vi "Parse OSZICAR (Energies).vi"(8 "error in (no error)":errorcluster, 9 "Reference Energy/atom (pure Crystal) (eV)":dbl=-2.489625, 10 "# of Atoms":i32, 11 "OSZICAR File":path) -> (0 "Summary Values":string[](array[string])=["# Atoms", "Cell Volume (A^3)", "|C|"], 1 "Summary Headers":string[](array[string])=["# Atoms", "Cell Volume (A^3)", "|A| (Å)", "|B| (Å)", "|C| (Å)", "alpha (deg)", "beta (deg)", "gamma (deg)"], 2 "OSZICAR Raw":T1, 3 "Extracted Parameters":T3)   [LabVIEW 2010]
panel:
  out "OSZICAR data":T2(array[cluster]) {"Total Free Energy (eV)" format="%#_10g"}
  out "error out":errorcluster
  out "Bulk Formation Energies Array (eV)":dbl[](array[numeric])
  out "Ionic Relaxation Energies Array (eV)":dbl[](array[numeric])
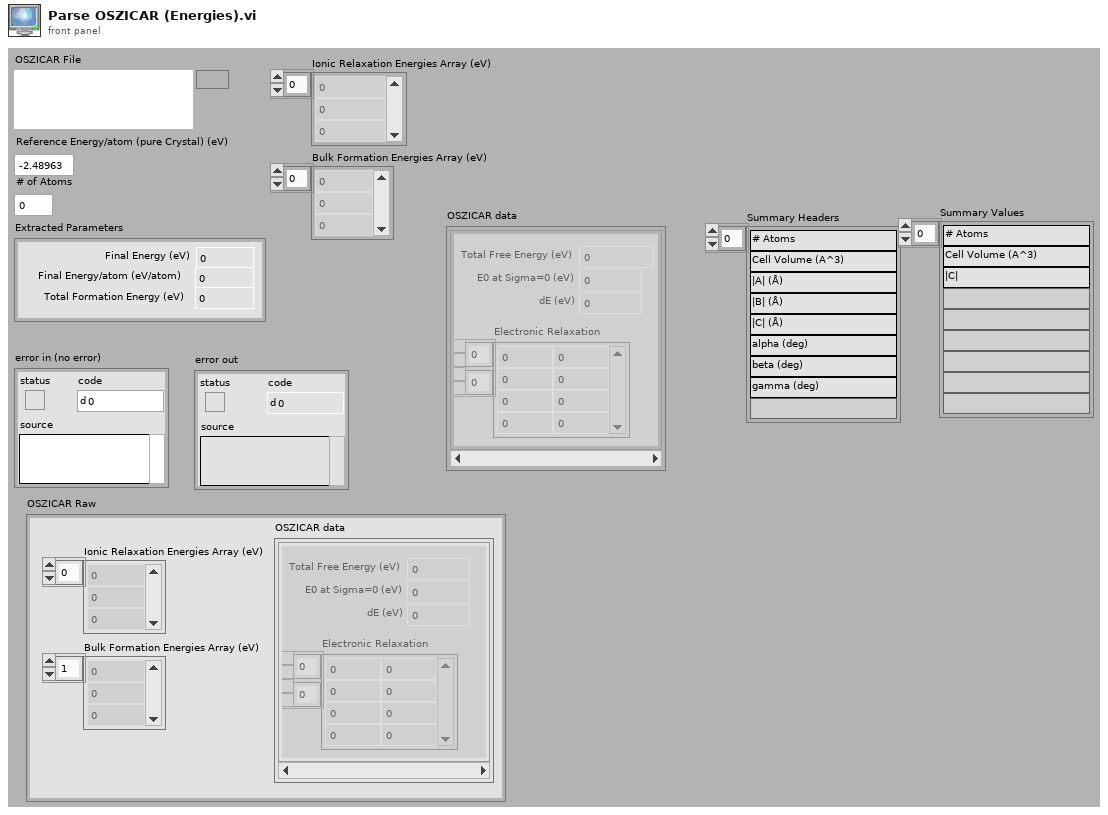
[diagram p1: front panel]
types:
  T1 = cluster{"OSZICAR data":cluster{"Total Free Energy (eV)":dbl, "E0 at Sigma=0 (eV)":dbl, "dE (eV)":dbl, "Electronic Relaxation":dbl[][]}[], "Ionic Relaxation Energies Array (eV)":dbl[], "Bulk Formation Energies Array (eV)":dbl[]}
  T2 = cluster{"Total Free Energy (eV)":dbl, "E0 at Sigma=0 (eV)":dbl, "dE (eV)":dbl, "Electronic Relaxation":dbl[][]}[]
  T3 = cluster{"Final Energy (eV)":dbl, "Final Energy/atom (eV/atom)":dbl, "Total Formation Energy (eV)":dbl}
  T4 = cluster{"Total Free Energy (eV)":dbl, "E0 at Sigma=0 (eV)":dbl, "dE (eV)":dbl, "Electronic Relaxation":dbl[][]}
  T5 = cluster{"OSZICAR data 2":cluster{"Total Free Energy (eV)":dbl, "E0 at Sigma=0 (eV)":dbl, "dE (eV)":dbl, "Electronic Relaxation":dbl[][]}[], dbl[], dbl[]}
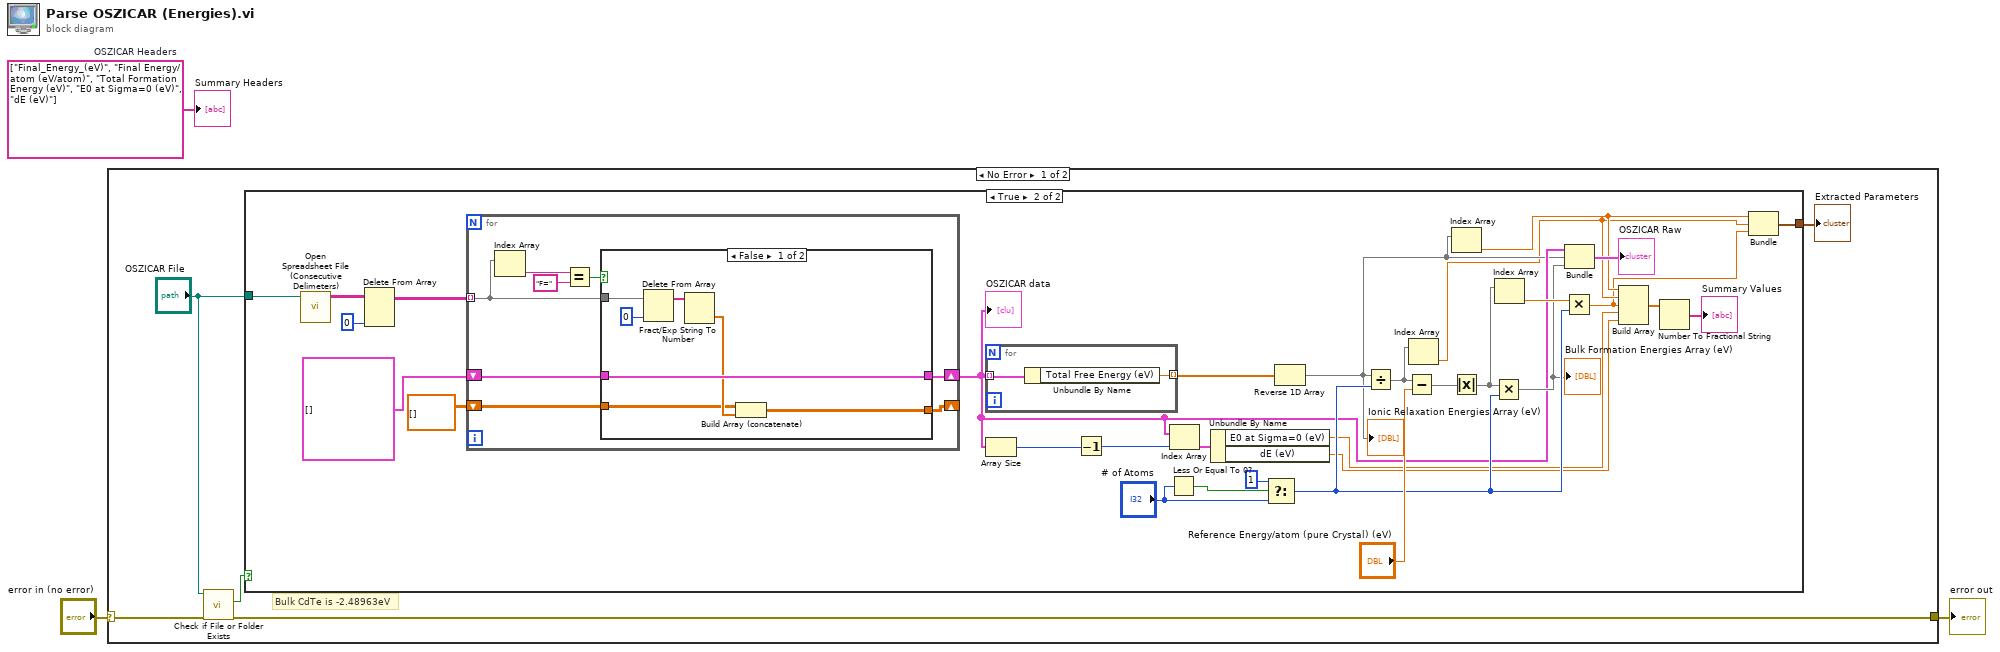
[diagram p0: block diagram]
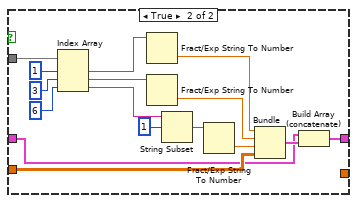
[diagram p3: hidden frame]
diagram:
  w1 = string[] ["Final_Energy_(eV)", "Final Energy/atom (eV/atom)", "Total Formation Energy (eV)", "E0 at Sigma=0 (eV)", "dE (eV)"]  # OSZICAR Headers
  n1 = case shown="No Error" "error in (no error)" {
    selector: "error in (no error)" -> [w5 w73]
    tunnel: [w4 w73] -> w2
    frame No Error {
      # "Bulk CdTe is -2.48963eV"
      n2 = call <vilib>:"Check if File or Folder Exists.vi"("error in (no error)"=w5, "path"="OSZICAR File") -> ("error out"=w4:errorcluster, "file or folder exists?"=w7:bool)  [unwired: 7 in, 1 out]
      n3 = case shown="True" w7 {
        tunnel: "OSZICAR File" -> [_ w29]
        tunnel: [_ w30] -> w6
        frame False {
        }
        frame True {
          n4 = call "Open Spreadsheet File (Consecutive Delimeters).vi"("File"=w29) -> ("Array"=w28:string[][])  [unwired: 9 in, 1 out]
          n5 = Delete From Array(array=w28, index (col)=0 ("disabled index (col)")) -> (array with subset deleted=w26:string[][])  [unwired: 2 in, 1 out]
          n6 = for {
            tunnel: w26 -> [w46] mode=indexing
            shift-right: [w45] -> _
            shift-left: dbl[][] [] -> [w44]
            shift-right: [w43] -> w20
            shift-left: T2 [] ("OSZICAR data 2") -> [w42]
            n7 = Index Array(array=w46) -> (element=w49:string)  [unwired: 1 in]
            n8 = Equal?(x=w49, y="F=") -> (x = y?=w47:bool)
            n9 = case shown="False" w47 {
              tunnel: w46 -> [w55 w64]
              tunnel: [w51 _] -> w45
              tunnel: w44 -> [w50 w69]
              tunnel: [w56 w67] -> w43
              tunnel: w42 -> [w56 w66]
              frame False {
                n10 = Delete From Array(array=w55, index=0) -> (array with subset deleted=w53:string[])  [unwired: 1 in, 1 out]
                n11 = Fract/Exp String To Number(string=w53) -> (number=w52:dbl[])  [unwired: 3 in, 1 out]
                n12 = Build Array (concatenate)(w50, w52) -> (w51:dbl[][])
              }
              frame True {
                n13 = Index Array(array=w64, index #1=1 ("index"), index #2=3 ("index"), index #3=6 ("index")) -> (element #1=w63:string, element #2=w61:string, element #3=w59:string)
                n14 = Fract/Exp String To Number(string=w63) -> (number=w62:dbl)  [unwired: 3 in, 1 out]
                n15 = Fract/Exp String To Number(string=w61) -> (number=w60:dbl)  [unwired: 3 in, 1 out]
                n16 = String Subset(string=w59, offset (0)=1) -> (substring=w58:string)  [unwired: 1 in]
                n17 = Fract/Exp String To Number(string=w58) -> (number=w57:dbl)  [unwired: 3 in, 1 out]
                n18 = Bundle(w62, w60, w57, w69) -> (w68:cluster{dbl, dbl, dbl, dbl[][]})  [unwired: 1 in]
                n19 = Build Array (concatenate)(w66, w68) -> (w67:T2)
              }
            }
          }
          "OSZICAR data" <- w20
          n20 = for {
            tunnel: w20 -> [w41] mode=indexing
            tunnel: [w40] -> w23 mode=indexing
            n21 = Unbundle By Name(w41) -> ("Total Free Energy (eV)"=w40:dbl)
          }
          n22 = Array Size(array=w20) -> (size(s)=w19:i32)
          n23 = Decrement(x=w19) -> (x-1=w18:i32)
          n24 = Less Or Equal To 0?(x="# of Atoms") -> (x <= 0?=w36:bool)
          n25 = Index Array(array=w20, index=w18) -> (element=w17:T4)
          n26 = Unbundle By Name(w17) -> ("E0 at Sigma=0 (eV)"=w16:dbl, "dE (eV)"=w15:dbl)
          n27 = Select(t=1, s=w36, f="# of Atoms") -> (s? t:f=w32:i32)
          n28 = Reverse 1D Array(array=w23) -> (reversed array=w14:dbl[])
          "Ionic Relaxation Energies Array (eV)" <- w14
          n29 = Divide(x=w14, y=w32) -> (x/y=w31:dbl[])
          n30 = Subtract(x=w31, y="Reference Energy/atom (pure Crystal) (eV)") -> (x-y=w38:dbl[])
          n31 = Index Array(array=w31) -> (element=w12:dbl)  [unwired: 1 in]
          n32 = Index Array(array=w14) -> (element=w13:dbl)  [unwired: 1 in]
          n33 = Absolute Value(x=w38) -> (abs(x)=w33:dbl[])
          n34 = Multiply(x=w33, y=w32) -> (x*y=w22:dbl[])
          "Bulk Formation Energies Array (eV)" <- w22
          n35 = Index Array(array=w33) -> (element=w37:dbl)  [unwired: 1 in]
          n36 = Multiply(x=w37, y=w32) -> (x*y=w11:dbl)
          n37 = Bundle("OSZICAR data 2"=w20, w14, w22) -> (→"OSZICAR Raw":T5)  [unwired: 1 in]
          n38 = Build Array(w13, w12, w11, w16, w15) -> (w10:dbl[])
          n39 = Number To Fractional String(number=w10) -> (F-format string=→"Summary Values":string[])  [unwired: 3 in]
          n40 = Bundle("Total Free Energy (eV)"=w13, w12, w11) -> (w30:cluster{"Total Free Energy (eV)":dbl, dbl, dbl})  [unwired: 1 in]
        }
      }
      "Extracted Parameters" <- w6
    }
    frame Error {
    }
  }
  "error out" <- w2
  "Summary Headers" <- w1
